vi "d.vi"(8 "error in (no error)":errorcluster, 11 "Arduino in":refnum<class "Arduino.lvclass">) -> (0 "error out":errorcluster, 2 "Serial Device Brand":T1, 3 "Arduino out":refnum<class "Arduino.lvclass">)   [LabVIEW 2019]
uses:
  Serial Device.lvclass
  Arduino.lvclass
  E:/7to semestre/instrumentacion virtual/proyecto final/proyecto-final/Serial Device.lvclass
  Control 13.ctl
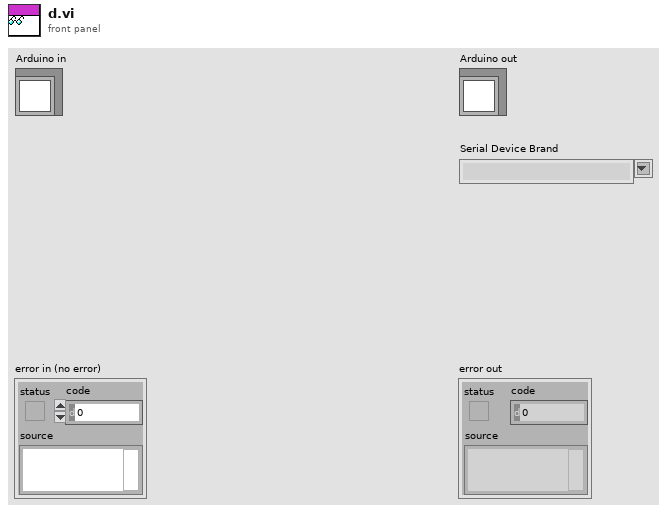
[diagram p1: front panel]
types:
  T1 = typedef "Serial Device.lvclass/Control 13.ctl" = string
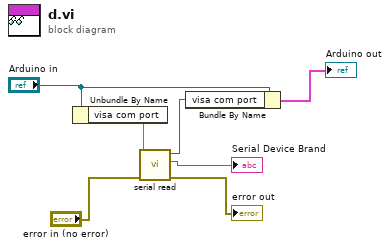
[diagram p0: block diagram]
diagram:
  n1 = Unbundle By Name("Arduino in") -> ("visa com port"=w7)
  n2 = call "serial read.vi"("error in (no error)"="error in (no error)", "VISA resource name"=w7) -> ("error out"=→"error out":errorcluster, "respuesta serial"=→"Serial Device Brand":string, "VISA resource nameout"=w4:refnum<visa-resource-name>)  [unwired: 7 in]
  n3 = Bundle By Name(cluster="Arduino in", "visa com port"=w4) -> (→"Arduino out":cluster{})
